vi "添加URL.vi"(8 "error in (no error)":errorcluster caption="错误输入（无错误）", 10 "URL":string="URL", 11 "簇":cluster{"URL":string}={"URL"="平台数据发送系统"}) -> (0 "error out":errorcluster caption="错误输出", 3 "添加成功标记":bool)   [LabVIEW 2016, in "数据传输系统-05.lvlib"]
uses:
  <vilib>/registry/registry.llb/Registry RtKey.ctl
  <vilib>/registry/registry.llb/Write Registry Value Simple STR.vi
panel:
  out "值":string[](array[string])
  out "名称":string[](array[string])
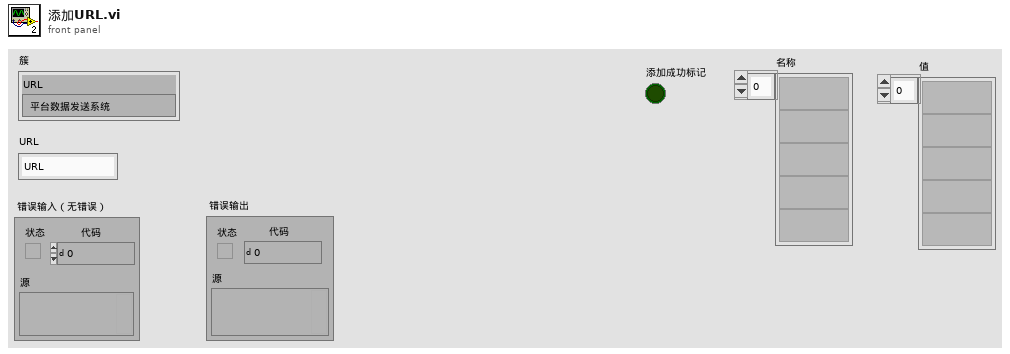
[diagram p1: front panel]
types:
  T1 = typedef "Registry RtKey.ctl" = enum32{"HKEY_CLASSES_ROOT", "HKEY_CURRENT_USER", "HKEY_LOCAL_MACHINE", "HKEY_USERS", "HKEY_PERFORMANCE_DATA", "HKEY_CURRENT_CONFIG", "HKEY_DYN_DATA"}
  T2 = typedef "Registry refnum.ctl" = refnum<k1>
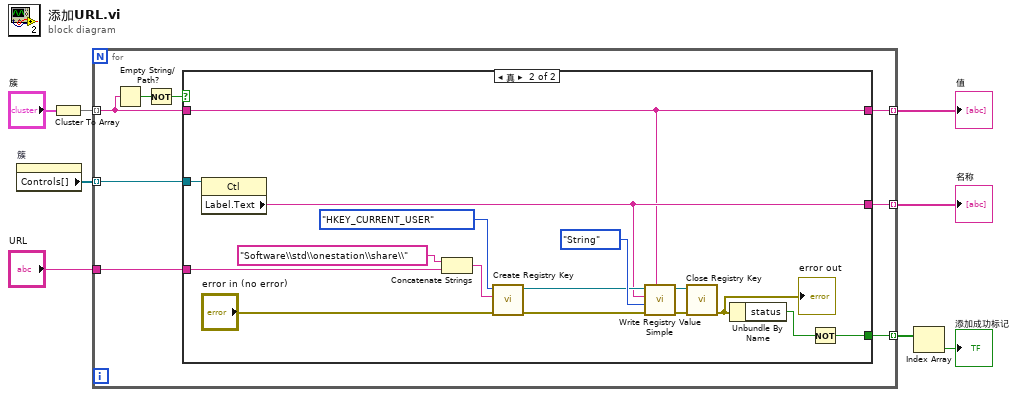
[diagram p0: block diagram]
diagram:
  n1 = property on="簇" class="Clust (严格)"() -> ("Controls[]"=w6:refnum<vi>[])  [unwired: 2 in, 2 out]
  n2 = Cluster To Array(cluster="簇") -> (array=w7:string[])
  n3 = for {
    tunnel: w7 -> [w14] mode=indexing
    tunnel: w6 -> [w13] mode=indexing
    tunnel: [w12] -> w5 mode=indexing
    tunnel: [w11] -> w4 mode=indexing
    tunnel: [w10] -> w3 mode=indexing
    tunnel: "URL" -> [w9]
    n4 = Empty String/Path?(string/path=w14) -> (empty?=w16:bool)
    n5 = Not(x=w16) -> (.not. x?=w15:bool)
    n6 = case shown="真" w15 {
      tunnel: w14 -> [_ w19]
      tunnel: [_ w27] -> w10
      tunnel: w13 -> [_ w21]
      tunnel: [_ w20] -> w12
      tunnel: [_ w19] -> w11
      tunnel: w9 -> [_ w17]
      frame False {
      }
      frame True {
        n7 = property class="Ctl"(reference=w21) -> ("Label.Text"=w20:string)  [unwired: 1 in, 2 out]
        n8 = Concatenate Strings("Software\\std\\onestation\\share\\" ("subkey"), w17) -> (w18:string)
        n9 = call <vilib>:"Create Registry Key.vi"("error in (no error)"="error in (no error)", "subkey"=w18, "root key (HKEY_LOCAL_MACHINE)"=Registry_RtKey."HKEY_CURRENT_USER") -> ("error out"=w23:errorcluster, "refnum out"=w24:T2)  [unwired: 6 in, 1 out]
        n10 = call-poly <vilib>:"Write Registry Value Simple.vi"("String/Binary data"=w19, "error in (no error)"=w23, "simple data type"=enum16{"String", "Binary", "DWORD"}."String", "value"=w20, "refnum"=w24) -> ("error out"=w32:errorcluster, "refnum out"=w31:T2)  [unwired: 3 in]
        n11 = call <vilib>:"Close Registry Key.vi"("error in (no error)"=w32, "refnum"=w31) -> ("error out"=w29:errorcluster)  [unwired: 5 in]
        "error out" <- w29
        n12 = Unbundle By Name(w29) -> ("status"=w28:bool)
        n13 = Not(x=w28) -> (.not. x?=w27:bool)
      }
    }
  }
  "名称" <- w5
  "值" <- w4
  n14 = Index Array(array=w3) -> (element=→"添加成功标记":bool)  [unwired: 1 in]
